vi "Write vi reference.vi"(8 "error in (no error)":errorcluster, 10 "vi reference":refnum<vi>, 11 "Oscilloscope in":refnum<class "Oscilloscope.lvclass">) -> (0 "error out":errorcluster, 3 "Oscilloscope out":refnum<class "Oscilloscope.lvclass">)   [LabVIEW 2018, in "Oscilloscope.lvclass"]
uses:
  Oscilloscope.lvclass
  Oscilloscope.lvclass/Oscilloscope.ctl
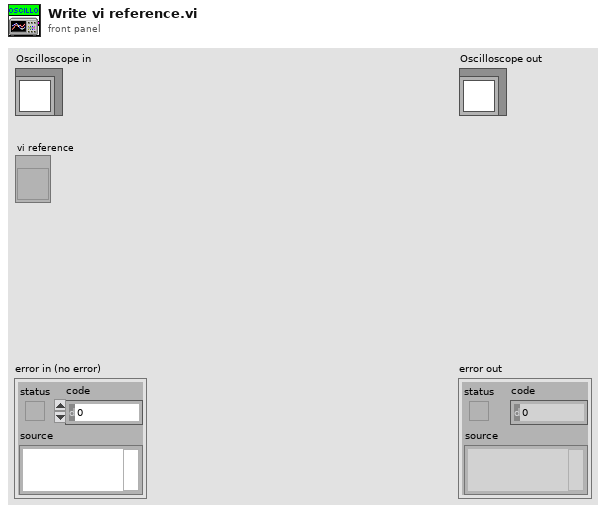
[diagram p1: front panel]
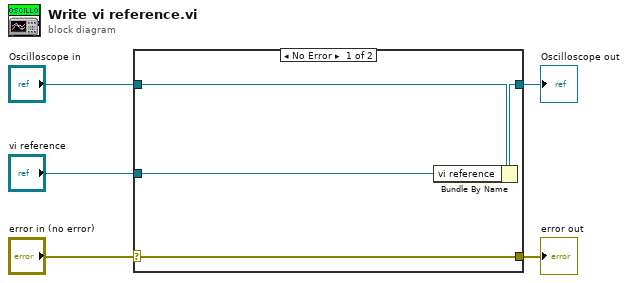
[diagram p0: block diagram]
diagram:
  n1 = case shown="No Error" "error in (no error)" {
    selector: "error in (no error)" -> [w9 w10]
    tunnel: [w9 w10] -> w4
    tunnel: [w7 w11] -> w2
    tunnel: "Oscilloscope in" -> [w8 w11]
    tunnel: "vi reference" -> [w6 _]
    frame No Error {
      n2 = Bundle By Name(cluster=w8, "vi reference"=w6) -> (w7:refnum<class "Oscilloscope.lvclass">)
    }
    frame Error {
    }
  }
  "error out" <- w4
  "Oscilloscope out" <- w2
